vi "Unflatten Value.vi"(8 "Error In":errorcluster, 10 "Value":string, 11 "TD Error Cluster In":refnum<class "Error Cluster.lvclass">) -> (0 "Error Out":errorcluster, 3 "TD Error Cluster Out":refnum<class "Error Cluster.lvclass">)   [LabVIEW 2017, in "Tree API.lvlib" / "Error Cluster.lvclass"]
doc: "Dynamic dispatch interface for unflattening Tree Data classes from string."
uses:
  Error Cluster.lvclass
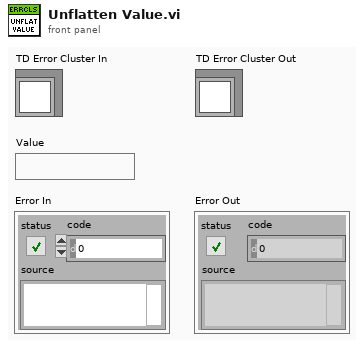
[diagram p1: front panel]
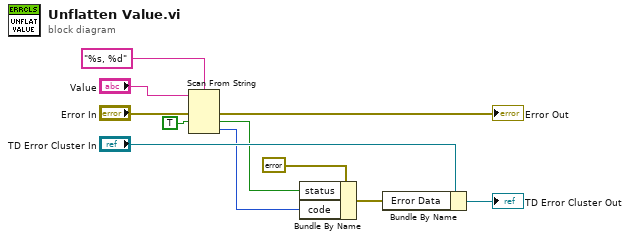
[diagram p0: block diagram]
diagram:
  n1 = Scan From String(format string="%s, %d", input string="Value", error in="Error In", default 1=TRUE) -> (error out=→"Error Out":errorcluster, output 1=w5:bool, output 2=w4:i32)  [unwired: 2 in, 2 out]
  n2 = Bundle By Name(cluster=errorcluster {"status"=FALSE, "code"=0, "source"=""} ("Error Data"), "status"=w5, "code"=w4) -> (w3:errorcluster)
  n3 = Bundle By Name(cluster="TD Error Cluster In", "Error Data"=w3) -> (→"TD Error Cluster Out":refnum<class "Error Cluster.lvclass">)
